vi "AIFIFORT.vi"(1 "AIsNamen":string[](array[string]), 2 "FPGA VI Reference In":refnum<k20>) -> ()   [LabVIEW 2010]
uses:
  <vilib>/rvi/interface/nirviMethod/nirviMethod.xnode
  C:/Users/HAGAR-IV/Desktop/Zeugs/Johnny/pertrasgc fpga/fpga-programm-2.vi
  GVAbschalten.vi
  GVtdms.vi
  GVZeitZyklus.vi
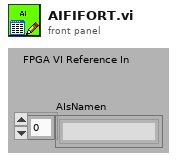
[diagram p1: front panel]
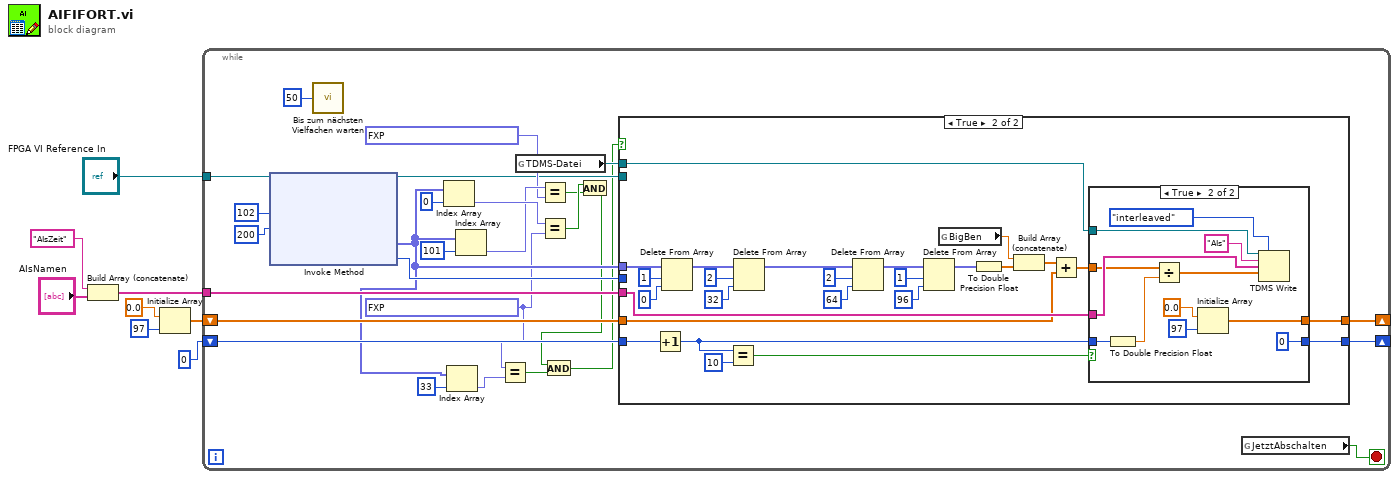
[diagram p0: block diagram]
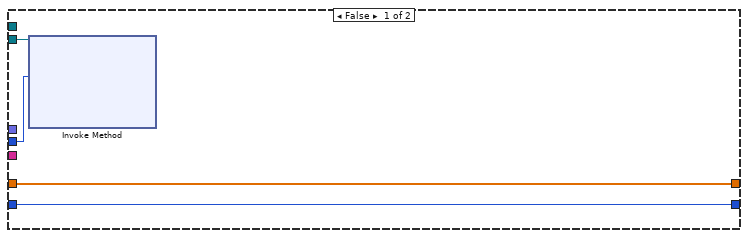
[diagram p2: hidden frame]
diagram:
  n1 = Build Array (concatenate)("AIsZeit", "AIsNamen") -> (w8:string[])
  n2 = Initialize Array(0.0 ("Element"), 97 ("Dimension")) -> (w4:dbl[])
  n3 = while {
    tunnel: "FPGA VI Reference In" -> [w23]
    tunnel: w8 -> [w25]
    shift-right: [w19] -> _
    shift-left: 0 -> [w21]
    shift-right: [w18] -> _
    shift-left: w4 -> [w20]
    stop <- w16 stop-if-true
    w12 = fxp<+/-,26,5> 1.0 ("y")
    n4 = xnode "Invoke Method"("FPGA VI Reference In"=w23, "Number of Elements"=u32 102, "Timeout (ms)"=200) -> ("FPGA VI Reference Out"=w22:refnum<k20>, "Data"=w14:fxp<+/-,26,5>[], "Elements Remaining"=w24:u32)  [unwired: 1 in, 1 out]
    n5 = call "Bis zum nächsten Vielfachen warten"("Count(mSec)"=u32 50) -> ()  [unwired: 1 out]
    n6 = Index Array(array=w14, index=0 ("Index")) -> (element=w33:fxp<+/-,26,5>)
    n7 = Index Array(array=w14, index=33 ("Index")) -> (element=w13:fxp<+/-,26,5>)
    n8 = Index Array(array=w14, index=101 ("Index")) -> (element=w32:fxp<+/-,26,5>)
    n9 = Equal?(x=w12, y=w13) -> (x = y?=w11:bool)
    n10 = global read "GVtdms.vi" "TDMS-Datei"() -> (w17:refnum<k34>)
    n11 = Equal?(x=w32, y=fxp<+/-,26,5> 3.0) -> (x = y?=w29:bool)
    n12 = Equal?(x=w33, y=w12) -> (x = y?=w30:bool)
    n13 = And(x=w30, y=w29) -> (x .and. y?=w10:bool)
    n14 = And(x=w10, y=w11) -> (x .and. y?=w9:bool)
    n15 = case shown="True" w9 {
      tunnel: w14 -> [_ w65]
      tunnel: w17 -> [_ w53]
      tunnel: w25 -> [_ w51]
      tunnel: w24 -> [w38 _]
      tunnel: w22 -> [w39 _]
      tunnel: w21 -> [w36 w50]
      tunnel: w20 -> [w37 w49]
      tunnel: [w36 w45] -> w19
      tunnel: [w37 w44] -> w18
      frame False {
        n16 = xnode "Invoke Method"("FPGA VI Reference In"=w39, "Number of Elements"=w38) -> ()  [unwired: 2 in, 4 out]
      }
      frame True {
        n17 = Increment(x=w50) -> (x+1=w46:i32)
        n18 = Delete From Array(array=w65, length=1 ("Länge"), index=0 ("Index")) -> (array with subset deleted=w60:fxp<+/-,26,5>[])  [unwired: 1 out]
        n19 = Equal?(x=w46, y=10) -> (x = y?=w48:bool)
        n20 = Delete From Array(array=w60, length=2 ("Länge"), index=32 ("Index")) -> (array with subset deleted=w57:fxp<+/-,26,5>[])  [unwired: 1 out]
        n21 = Delete From Array(array=w57, length=2 ("Länge"), index=64 ("Index")) -> (array with subset deleted=w54:fxp<+/-,26,5>[])  [unwired: 1 out]
        n22 = Delete From Array(array=w54, length=1 ("Länge"), index=96 ("Index")) -> (array with subset deleted=w52:fxp<+/-,26,5>[])  [unwired: 1 out]
        n23 = global read "GVZeitZyklus.vi" "BigBen"() -> (w42:dbl)
        n24 = To Double Precision Float(number=w52) -> (double precision float=w43:dbl[])
        n25 = Build Array (concatenate)(w42, w43) -> (w41:dbl[])
        n26 = Add(x=w41, y=w49) -> (x+y=w47:dbl[])
        n27 = case shown="True" w48 {
          tunnel: w53 -> [_ w79]
          tunnel: w51 -> [_ w77]
          tunnel: w47 -> [w67 w75]
          tunnel: w46 -> [w66 w74]
          tunnel: [w66 0] -> w45
          tunnel: [w67 w68] -> w44
          frame False {
          }
          frame True {
            n28 = To Double Precision Float(number=w74) -> (double precision float=w73:dbl)
            n29 = Divide(x=w75, y=w73) -> (x/y=w72:dbl[])
            n30 = Initialize Array(0.0 ("Element"), 97 ("Dimension")) -> (w68:dbl[])
            n31 = TDMS Write(0:w79, 1:enum16{"decimated", "interleaved"}."interleaved" ("Daten-Layout (0:dezimiert)"), 5:"AIs" ("Gruppenname (Eingang, Unbenannt)"), 7:w77, 9:w72) -> ()  [unwired: 1 in, 4 out]
          }
        }
      }
    }
    n32 = global read "GVAbschalten.vi" "JetztAbschalten"() -> (w16:bool)
  }
